vi "Configure Jitter Measurement (+Width to +Width).vi"(8 "error in (no error)":errorcluster, 10 "Source +Width to +Width (0: Channel 1)":u16(ring) items=["Channel 1", "Channel 2", "Channel 3", "Channel 4", "Math 1", "Math 2", "Math 3", "Math 4", "Reference Waveform 1", "Reference Waveform 2", "Reference Waveform 3", "Reference Waveform 4"], 11 "VISA resource name":refnum<visa-resource-name>) -> (0 "error out":errorcluster, 3 "VISA resource name out":refnum<visa-resource-name>)   [LabVIEW 2016, in "Agilent 2000 3000 X-Series.lvlib"]
doc: "Enables Jitter Analysis and configure the +Width to +Width (cycle-to-cycle positive width) jitter measurement. The +Width to +Width jitter measurement subtracts the first cycle's positive pulse width from the second cycle's positive pulse width for the first measurement result. Then, the second cycle's positive pulse width is subtracted from the third cycle's positive pulse width for the second measurement result, and so on, until all of the cycles of the waveform have been measured.\n\n<b>Note:</b>\nThis VI is specific to the 6000-X Series oscilloscopes. These features are not available on other models."
uses:
  Agilent 2000 3000 X-Series.lvlib
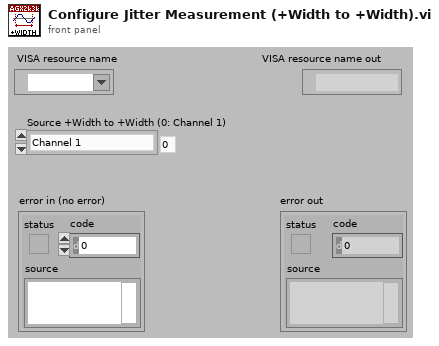
[diagram p1: front panel]
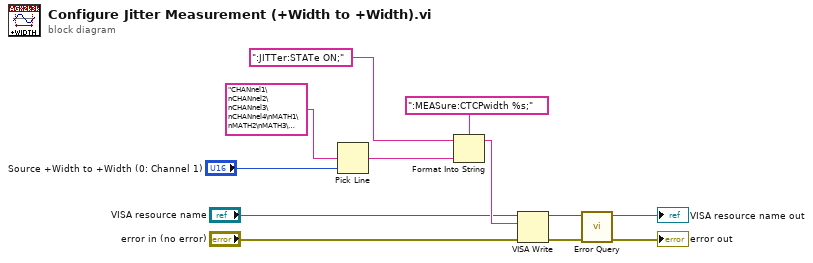
[diagram p0: block diagram]
diagram:
  n1 = Pick Line(multi-line string="CHANnel1\nCHANnel2\nCHANnel3\nCHANnel4\nMATH1\nMATH2\nMATH3\nMATH4\nWMEMory1\nWMEMory2\nWMEMory3\nWMEMory4", line index="Source +Width to +Width (0: Channel 1)") -> (output string=w10:string)  [unwired: 1 in]
  n2 = Format Into String(format string=":MEASure:CTCPwidth %s;", initial string=":JITTer:STATe ON;", w10) -> (resulting string=w7:string)  [unwired: 1 in, 1 out]
  n3 = VISA Write(VISA resource name="VISA resource name", write buffer=w7, error in (no error)="error in (no error)") -> (VISA resource name out=w9:refnum<visa-resource-name>, error out=w8:errorcluster)  [unwired: 1 out]
  n4 = call "Error Query.vi"("error in (no error)"=w8, "VISA resource name"=w9) -> ("error out"=→"error out":errorcluster, "VISA resource name out"=→"VISA resource name out":refnum<visa-resource-name>)  [unwired: 6 in, 2 out]
